vi "Test Tree.vi"() -> ()   [LabVIEW 2016]
uses:
  <vilib>/event_ctls.llb/eventsource.ctl
  <vilib>/event_ctls.llb/lveventtype.ctl
  <vilib>/Utility/miscctls.llb/LVPoint32TypeDef.ctl
  <vilib>/picture/picture.llb/imagedata.ctl
panel:
  out "image data 2":T1
  in  "mask":u8[](array[numeric])=[255, 255, 255]
  out "Custom Item Symbols:Get Symbol":T1
  out "image data":T1
  in  "path to PNG file":path=path "D:/github/Measure_core/Data/settings1_16x16.png"
  out "Click Tag":string="child 1"
  out "In Symbol?":bool
  out "error out":errorcluster
  out "NewVal":string="child 1"
  out "Tag":string="root"
  out "CellPart":T2(ring)=enum."Open/Close Symbol"
  out "PlatMods":T3
  out "Mods":cluster{"Double Click":bool, "Menu Key":bool}={"Double Click"=TRUE, "Menu Key"=FALSE}
  out "Button":u16=1
  out "Coords":T4={"Horizontal"=502, "Vertical"=-46}
  out "Type":T5=enum."Tree Double Click"
  out "Source":T6 items=["LabVIEW UI"=0, "ActiveX"=1, "User Event"=25]
  in  "Tree":string(tree)="child 2"
  in  "Array - Numeric":dbl[](array[numeric])
  in  "Stop Button":bool
  in  "Numeric Control":dbl
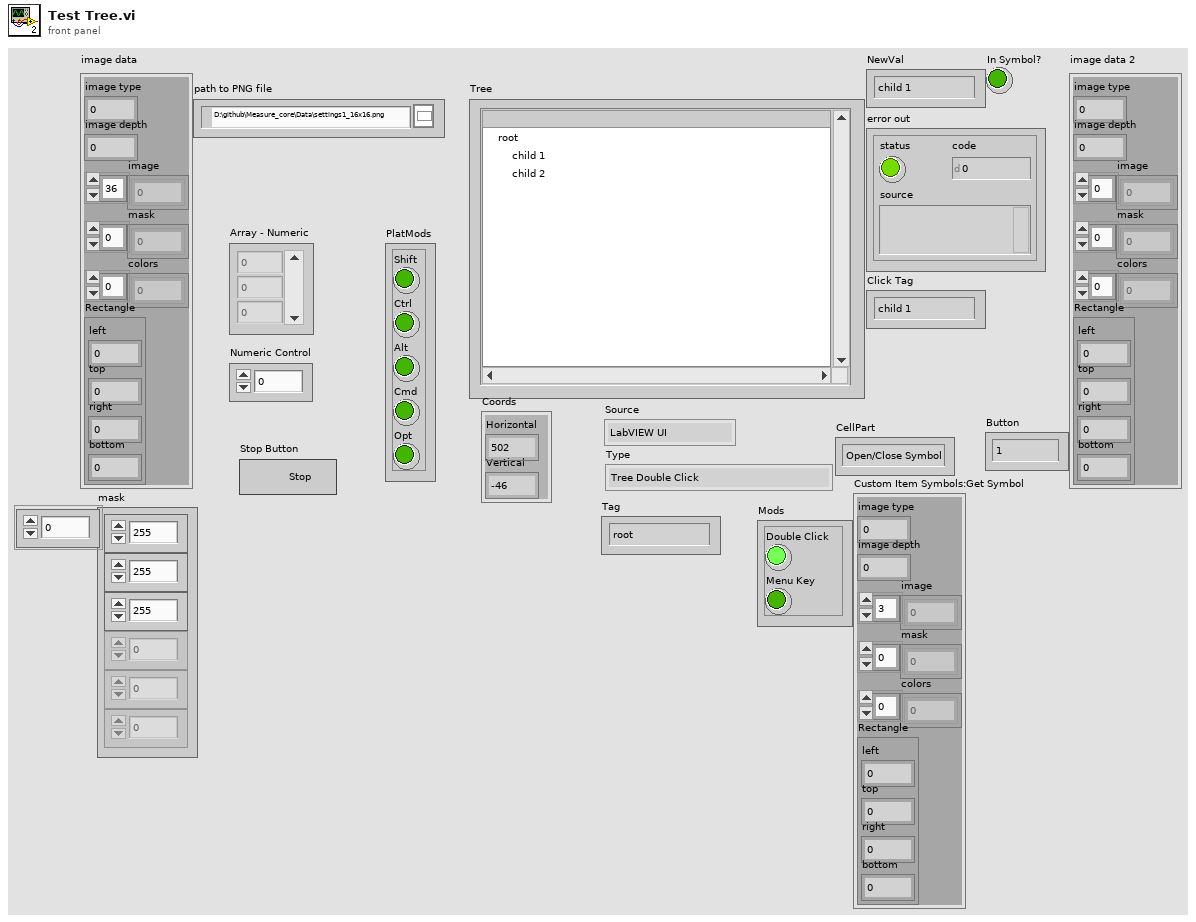
[diagram p1: front panel]
types:
  T1 = typedef "imagedata.ctl" = cluster{"image type":i32, "image depth":i32, "image":u8[], "mask":u8[], "colors":u32[], "Rectangle":cluster{"left":i16, "top":i16, "right":i16, "bottom":i16}}
  T2 = enum16{"Text", "Background", "Item Symbol", "Open/Close Symbol", "Hierarchy Lines", "Right Border", "Bottom Border", "Bottom Right Corner", "Unknown Part"}
  T3 = cluster{"Shift":bool, "Ctrl":bool, "Alt":bool, "Cmd":bool, "Opt":bool}
  T4 = typedef "LVPoint32TypeDef.ctl" = cluster{"Horizontal":i32, "Vertical":i32}
  T5 = typedef "lveventtype.ctl" = enum32{"Null", "Timeout", "Annotation Menu Selection", "Annotation Menu Selection?", "App Instance Close", "App Instance Close?", "Autoscale Range Change", "Bookmark Info Change", "Cell Edit", "Cell Edit?", "Cursor Grab", "Cursor Grab?", "Cursor Menu Selection", "Cursor Menu Selection?", "Cursor Move", "Cursor Release", "Data Change", "Direction Change", "Display State Change", "Drag Ended", "Drag Enter", "Drag Leave", "Drag Over", "Drag Source Update", "Drag Starting", "Drag Starting?", "Drop", "Exec State Change", "Key Down", "Key Down?", "Key Repeat", "Key Repeat?", "Key Up", "Listbox Double Click", "Menu Activation?", "Menu Selection (App)", "Menu Selection? (App)", "Menu Selection (User)", "Mouse Down", "Mouse Down?", "Mouse Enter", "Mouse Leave", "Mouse Move", "Mouse Up", "Mouse Wheel", "NI Security User Change (App)", "Pane Size", "Panel Close", "Panel Close?", "Panel Resize", "Plot Attribute Change", "Scale Range Change", "Shortcut Menu Activation?", "Shortcut Menu Selection (App)", "Shortcut Menu Selection? (App)", "Shortcut Menu Selection (User)", "Tree Double Click", "Tree Drag", "Tree Drag?", "Tree Drop", "Tree Drop?", "Tree Item Close", "Tree Item Close?", "Tree Item Open", "Tree Item Open?", "User Event", "Value Change"}
  T6 = typedef "eventsource.ctl" = u32
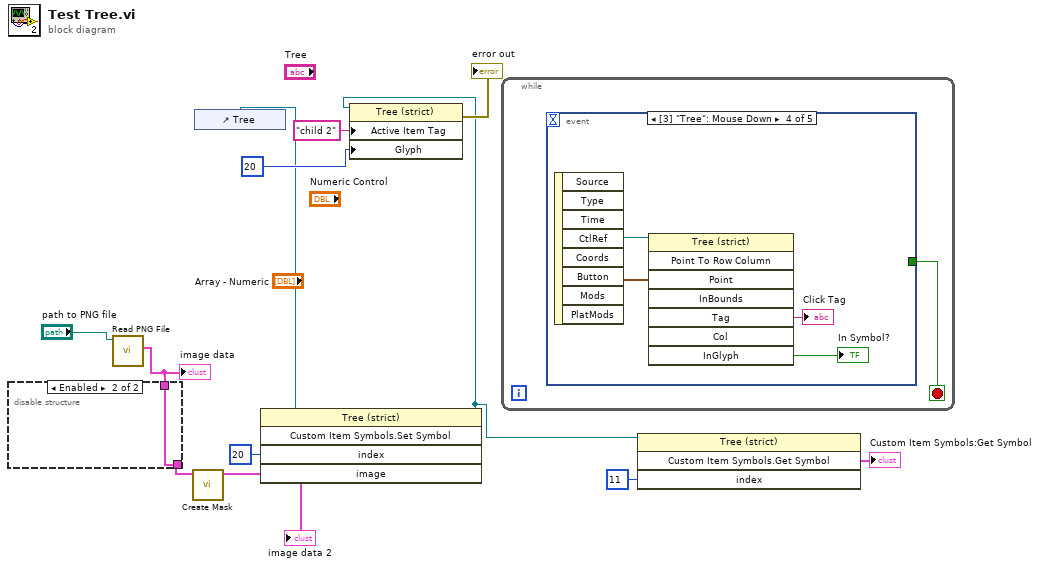
[diagram p0: block diagram]
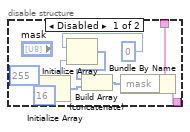
[diagram p2: hidden frame]
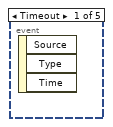
[diagram p3: hidden frame]
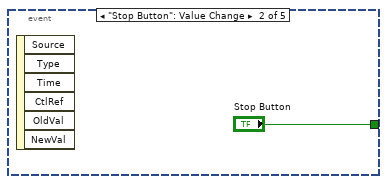
[diagram p4: hidden frame]
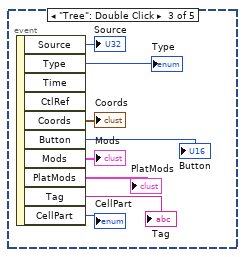
[diagram p5: hidden frame]
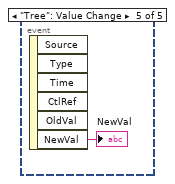
[diagram p6: hidden frame]
diagram:
  n1 = call <vilib>:"Read PNG File.vi"("path to PNG file"="path to PNG file") -> ("image data"=w6:T1)  [unwired: 8 in, 2 out]
  "image data" <- w6
  n2 = disable-structure shown="Enabled" {
    disable-tunnel: w6 -> [w20 w21]
    disable-tunnel: [w19 w21] -> w2
    frame Disabled {
      w15 = 16 ("dimension size")
      n3 = Initialize Array(u8 255, w15) -> (w17:u8[])
      n4 = Initialize Array(u8 0, w15) -> (w13:u8[])
      n5 = Build Array (concatenate)(w13, w17) -> (w16:u8[])
      n6 = Bundle By Name(cluster=w20, "mask"=w16) -> (w19:T1)
    }
    frame Enabled {
    }
  }
  n7 = call <vilib>:"Create Mask.vi"("image data"=w2) -> ("image data"=w1:T1)  [unwired: 10 in]
  "image data 2" <- w1
  n8 = control-ref of="Tree"() -> (w9:refnum<vi>)
  n9 = invoke class="Tree (strict)" method="Custom Item Symbols.Set Symbol"(reference=w9, "index"=20 ("Index"), "image"=w1) -> (reference out=w5:refnum<vi>)  [unwired: 2 in, 4 out]
  n10 = property class="Tree (strict)"(reference=w5, "Active Item Tag"="child 2" ("Active Item:Tag"), "Glyph"=20 ("Active Item:Symbol Index")) -> (error out=→"error out":errorcluster)  [unwired: 1 in, 1 out]
  n11 = while {
    stop <- w22 stop-if-true
    n12 = event shown="[3] \"Tree\": Mouse Down" {
      selector: _ -> [_ _ _ _ _]
      dyn-events: _ -> [_ _ _ _ _]
      timeout: _ -> [_ _ _ _ _]
      tunnel: [_ "Stop Button" _ _ _] -> w22
      event Timeout {
        n13 = event-data() -> ()  [unwired: 1 in, 3 out]
      }
      event "Stop Button": Value Change {
        n14 = event-data() -> ()  [unwired: 1 in, 6 out]
      }
      event "Tree": Double Click {
        n15 = event-data() -> ("Source"=→"Source":T6, "Type"=→"Type":T5, "Coords"=→"Coords":T4, "Button"=→"Button":u16, "Mods"=→"Mods":cluster{"Double Click":bool, "Menu Key":bool}, "PlatMods"=→"PlatMods":T3, "Tag"=→"Tag":string, "CellPart"=→"CellPart":T2)  [unwired: 1 in, 2 out]
      }
      event "Tree": Mouse Down {
        n16 = event-data() -> ("CtlRef"=w35:refnum<vi>, "Coords"=w34:T4)  [unwired: 1 in, 6 out]
        n17 = invoke class="Tree (strict)" method="Point To Row Column"(reference=w35, "Point"=w34) -> ("Tag"=→"Click Tag":string, "InGlyph"=→"In Symbol?":bool)  [unwired: 6 in, 6 out]
      }
      event "Tree": Value Change {
        n18 = event-data() -> ("NewVal"=→"NewVal":string)  [unwired: 1 in, 5 out]
      }
    }
  }
  n19 = invoke class="Tree (strict)" method="Custom Item Symbols.Get Symbol"(reference=w5, "index"=11) -> ("Custom Glyphs:Get Glyph"=→"Custom Item Symbols:Get Symbol":T1)  [unwired: 2 in, 3 out]
